vi "6-2-2.vi"() -> ()   [LabVIEW 2022 SP3, in "AoC22.lvlib"]
uses:
  AoC22.lvlib
panel:
  out "Numeric":i32
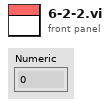
[diagram p1: front panel]
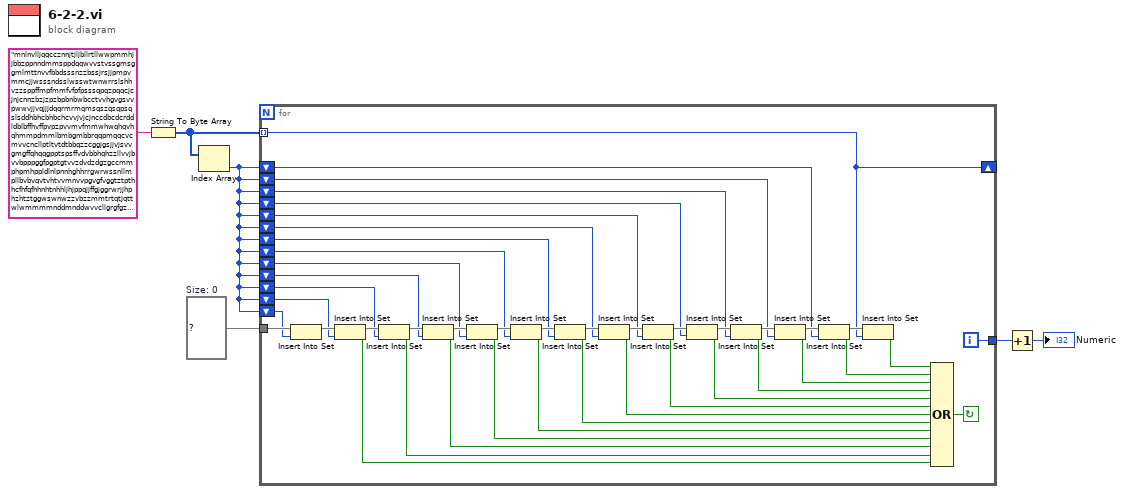
[diagram p0: block diagram]
diagram:
  w2 = set{u8} {}  # Size: 0
  n1 = String To Byte Array(string="mnlnvlljqqccznnjtjljbllrtllwwpmmhjjbbzppnndmmsppdqqwvvstvssgmsggmlmttnvvfbbdsssnzzbssjrsjjpmpvmmcjjwsssndsslwsswtwnwrrslshhvzzsppffmpfmmfvfpfpsssqpqzpqqcjcjnjcnnzbzjzpzbpbnbwbcctvvhgvgsvvpwwvjjvqjjjdqqrmrmqmsqszqsqpsqslsddhbhcbhbchcvvjvjcjnccdbcdcrddldblbffhvffpvpzpvvmvfmmwhwqhqvhqhmmpdmmlbmbgmbbrqqpmqqcvcmvvcncllptltvtdtbbqzzcggjgsjjvjsvvgmgffqhqqgpptspsffvdvbbhqhzzllvvjbvvbpppggfpgptgtvvzdvdzdgzgccmmphpmhppldlnlpnnhghhrrgwrwssnllmpllbvbvqvtvhtvvmnvvpgvgfvggtztpthhcfhfqfhhnhtnhhljhjppqjjffgjggrwrjjhphzhtztggwswnwzzvbzzmmtrtqtjqttwlwmmmmnddmnddwvvcllgrgfgzznwnsswjjhwwspsbbvzzqvzvbvcvmmtltnlnfn...") -> (unsigned byte array=w3:u8[])
  n2 = Index Array(array=w3) -> (element=w1:u8)  [unwired: 1 in]
  n3 = for {
    tunnel: w3 -> [w17] mode=indexing
    shift-right: [w17] -> _
    shift-left: w1 -> [w41]
    shift-left: w1 -> [w42]
    shift-left: w1 -> [w46]
    tunnel: [w48] -> w5
    tunnel: w2 -> [w47]
    shift-left: w1 -> [w16]
    shift-left: w1 -> [w15]
    shift-left: w1 -> [w14]
    shift-left: w1 -> [w13]
    shift-left: w1 -> [w12]
    shift-left: w1 -> [w11]
    shift-left: w1 -> [w10]
    shift-left: w1 -> [w9]
    shift-left: w1 -> [w8]
    shift-left: w1 -> [w7]
    i -> [w48]
    stop <- w49 continue-if-true
    n4 = Insert Into Set(10:w46, 11:w47) -> (3:w45:set{u8})  [unwired: 1 out]
    n5 = Insert Into Set(10:w42, 11:w45) -> (2:w40:bool, 3:w44:set{u8})
    n6 = Insert Into Set(10:w41, 11:w44) -> (2:w39:bool, 3:w43:set{u8})
    n7 = Insert Into Set(10:w16, 11:w43) -> (2:w38:bool, 3:w37:set{u8})
    n8 = Insert Into Set(10:w15, 11:w37) -> (2:w27:bool, 3:w36:set{u8})
    n9 = Insert Into Set(10:w14, 11:w36) -> (2:w26:bool, 3:w35:set{u8})
    n10 = Insert Into Set(10:w13, 11:w35) -> (2:w25:bool, 3:w34:set{u8})
    n11 = Insert Into Set(10:w12, 11:w34) -> (2:w24:bool, 3:w33:set{u8})
    n12 = Insert Into Set(10:w11, 11:w33) -> (2:w23:bool, 3:w32:set{u8})
    n13 = Insert Into Set(10:w10, 11:w32) -> (2:w22:bool, 3:w31:set{u8})
    n14 = Insert Into Set(10:w9, 11:w31) -> (2:w21:bool, 3:w30:set{u8})
    n15 = Insert Into Set(10:w8, 11:w30) -> (2:w20:bool, 3:w29:set{u8})
    n16 = Insert Into Set(10:w7, 11:w29) -> (2:w19:bool, 3:w28:set{u8})
    n17 = Insert Into Set(10:w17, 11:w28) -> (2:w18:bool)  [unwired: 1 out]
    n18 = Compound Arithmetic op=OR(w18, w19, w20, w21, w22, w23, w24, w25, w26, w27, w38, w39, w40) -> (w49:bool)
  }
  n19 = Increment(x=w5) -> (x+1=→"Numeric":i32)
